vi "Configure.vi"(8 "error in (no error)":errorcluster, 11 "GPIB In":refnum<visa-resource-name>) -> (0 "error out":errorcluster, 3 "GPIB Out":refnum<visa-resource-name>)   [LabVIEW 2015, in "Xitron 2503AH Library.lvlib"]
uses:
  Xitron 2503AH Library.lvlib
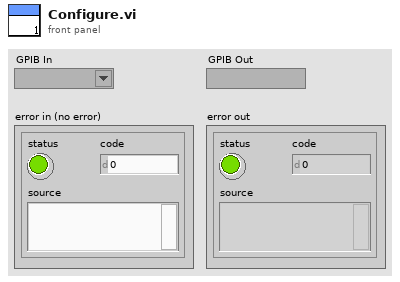
[diagram p1: front panel]
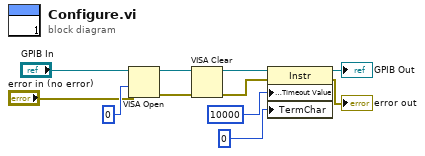
[diagram p0: block diagram]
diagram:
  n1 = VISA Open(access mode=u32 0, error in (no error)="error in (no error)", VISA resource name="GPIB In") -> (VISA resource name=w9:refnum<visa-resource-name>, error out=w8:errorcluster)  [unwired: 2 in]
  n2 = VISA Clear(VISA resource name=w9, error in (no error)=w8) -> (VISA resource name out=w7:refnum<visa-resource-name>, error out=w6:errorcluster)
  n3 = property class="Instr"(reference=w7, error in=w6, "General Settings:Timeout Value"=u32 10000, "TermChar"=u8 0 ("Message Based Settings:Termination Character")) -> (reference out=→"GPIB Out":refnum<visa-resource-name>, error out=→"error out":errorcluster)
